vi "Rotateable_i.vi"(1 "背景":u32[][](array[numeric]), 2 "point":cluster{"x":i16, "y":i16} caption="位置", 3 "编号":i8) -> (0 "Rotateable":bool)   [LabVIEW 2014]
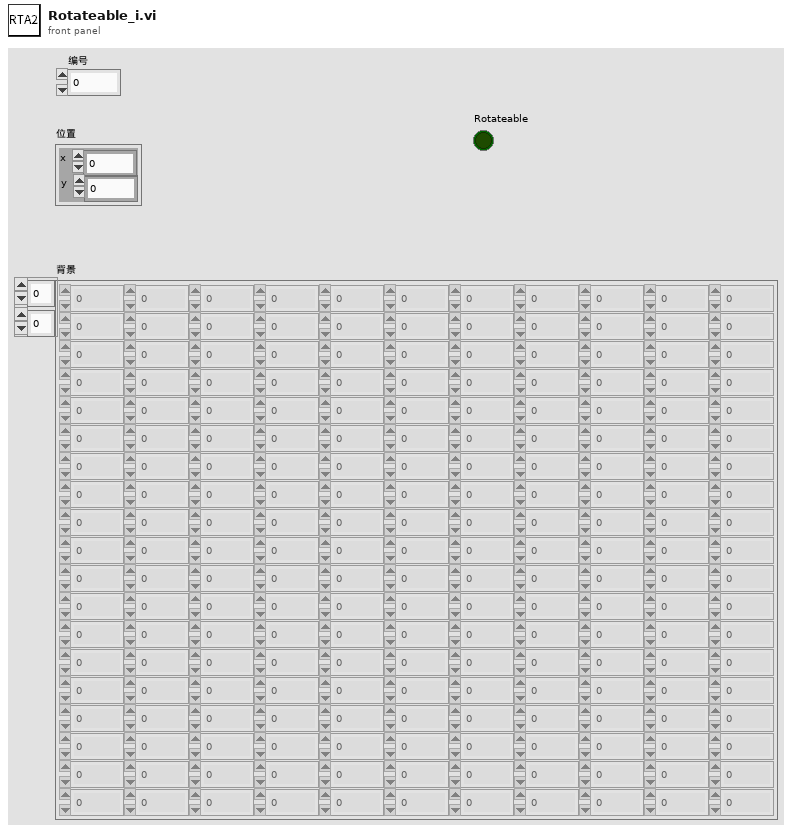
[diagram p1: front panel]
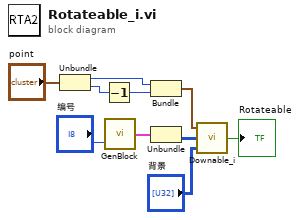
[diagram p0: block diagram]
diagram:
  n1 = Unbundle("point") -> ("x"=w4:i16, "y"=w5:i16)
  n2 = Decrement(x=w5) -> (x-1=w3:i16)
  n3 = call "GenBlock.vi"("编号"="编号") -> ("输出"=w9:cluster{"编号":i8, "方块":u32[][]})  [unwired: 1 in]
  n4 = Bundle("x"=w4, w3) -> (w2:cluster{"x":i16, i16})  [unwired: 1 in]
  n5 = Unbundle(w9) -> ("方块"=w8:u32[][])  [unwired: 1 out]
  n6 = call "Downable_i.vi"("背景"="背景", "方块"=w8, "point"=w2) -> ("输出"=→"Rotateable":bool)
